vi "HRV_EEG_version2.vi"() -> ()   [LabVIEW 2014]
uses:
  <vilib>/Utility/file.llb/Read From Spreadsheet File (I64).vi
panel:
  out "PPI+ERP":dbl[][](graph)
  out "HF+ERP":dbl[][](graph)
  out "LF+ERP":dbl[][](graph)
  out "VLF+ERP":dbl[][](graph)
  out "PPI":dbl[][](graph)
  in  "PPI":path=path "C:/Users/Jaehong/Desktop/Classifiers/HRV_EEG/LF Maker/김다영_PPI.txt"
  in  "HF":path=path "C:/Users/Jaehong/Desktop/Classifiers/HRV_EEG/LF Maker/김다영_HF.txt"
  in  "LF":path=path "C:/Users/Jaehong/Desktop/Classifiers/HRV_EEG/LF Maker/김다영_LF.txt"
  in  "VLF":path=path "C:/Users/Jaehong/Desktop/Classifiers/HRV_EEG/LF Maker/김다영_VLF.txt"
  in  "강제 Execution":bool
  out "HF":dbl[][](graph)
  out "LF":dbl[][](graph)
  out "VLF":dbl[][](graph)
  out "Executing":bool
  out "Target_icon":i64
  in  "Target_Total":path=path "C:/Users/Jaehong/Desktop/Classifiers/data/통합LDAs/김다영/target_order.txt"
  in  "Icon_number":i32=1
  out "ERP_Graph":dbl[][](graph)
  in  "Trial_Number":i32=1
  in  "ERP_Total":path=path "C:/Users/Jaehong/Desktop/Classifiers/HRV_EEG/ERP_total/김다영/ERP_total.txt"
  in  "stop":bool
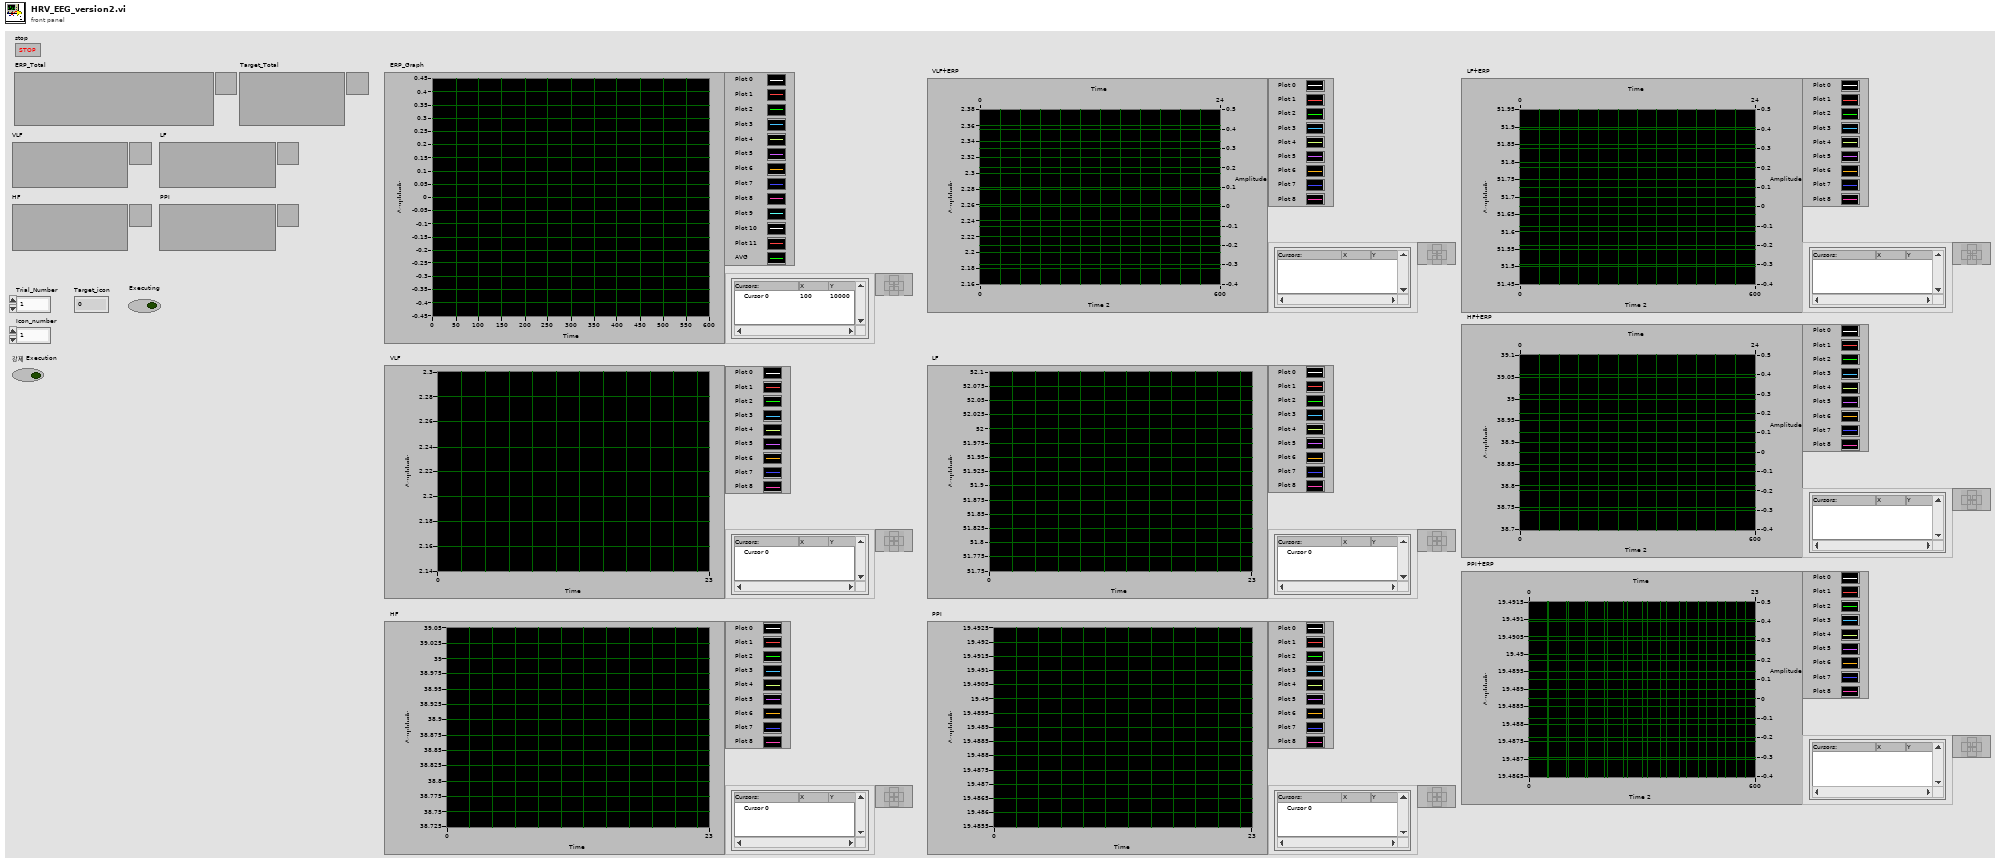
[diagram p1: front panel]
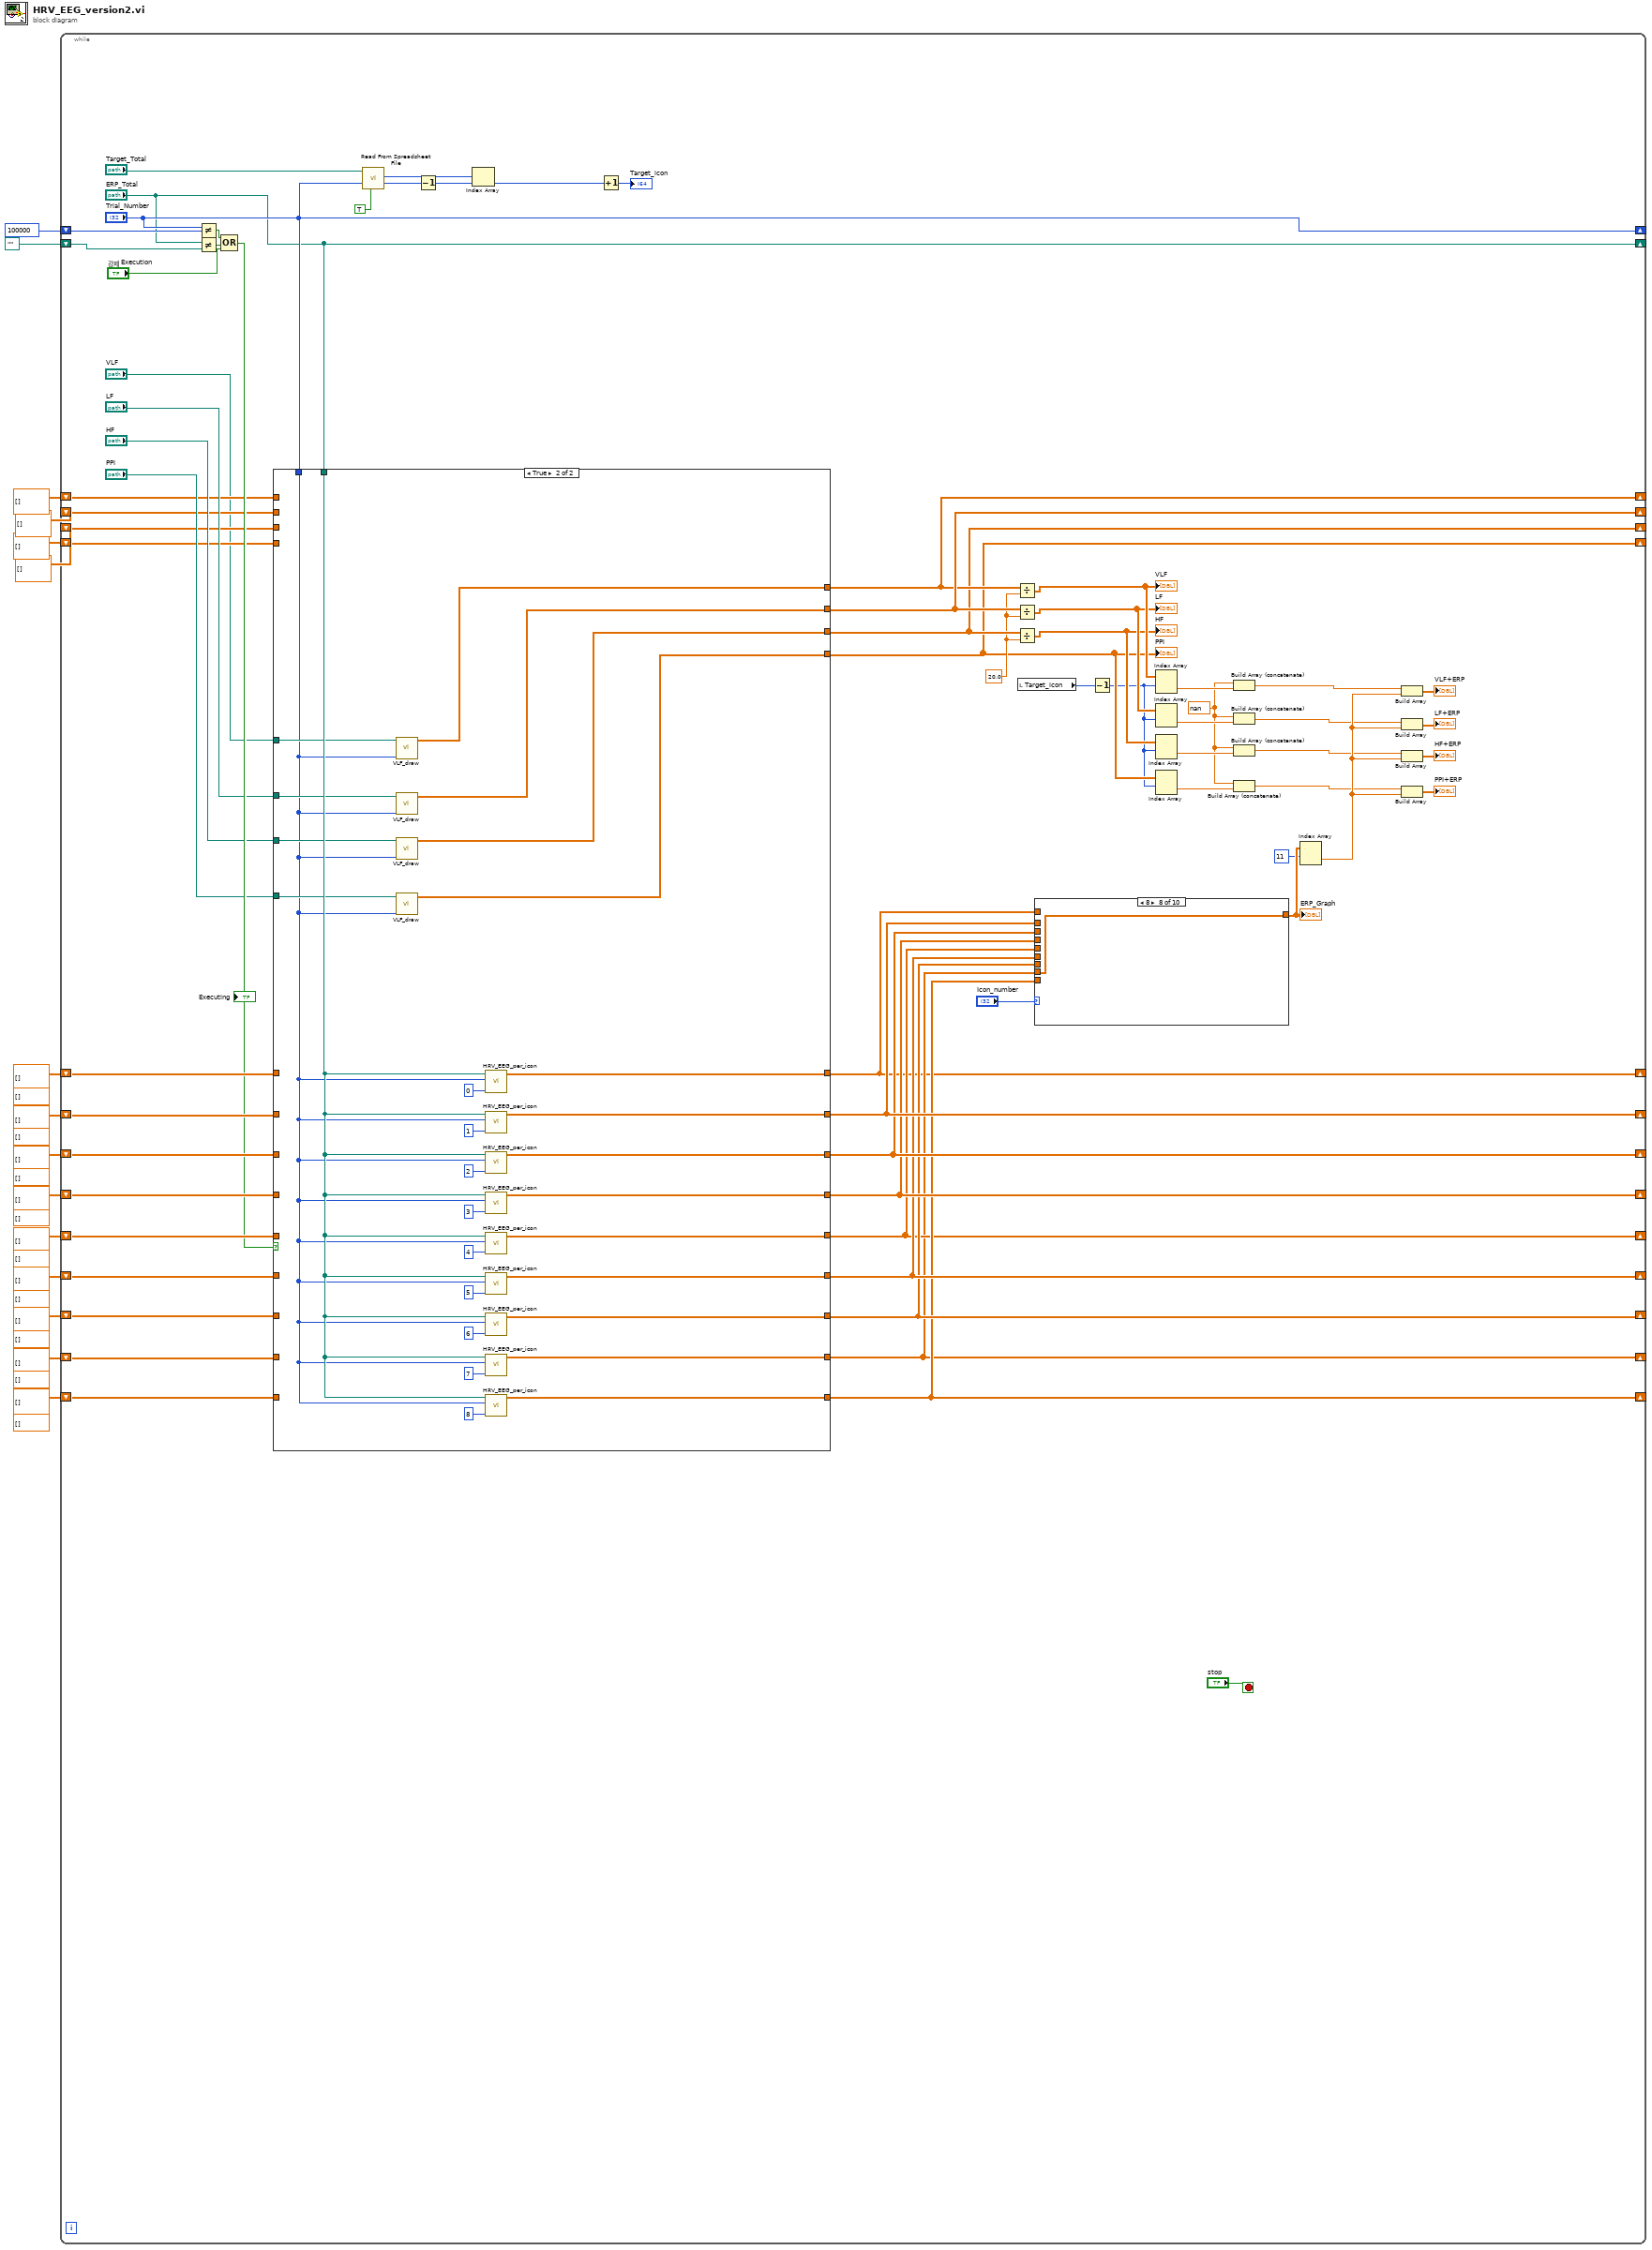
[diagram p0: block diagram]
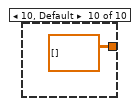
[diagram p11: hidden frame]
diagram:
  (unwired) dbl[] [] ("PRV% (VLF, LF, HF)")
  (unwired) dbl[] [] ("PRV% (VLF, LF, HF)")
  (unwired) dbl[] [] ("PRV% (VLF, LF, HF)")
  (unwired) dbl[] [] ("PRV% (VLF, LF, HF)")
  (unwired) dbl[] [] ("PRV% (VLF, LF, HF)")
  (unwired) dbl[] [] ("PRV% (VLF, LF, HF)")
  (unwired) dbl[] [] ("PRV% (VLF, LF, HF)")
  (unwired) dbl[] [] ("PRV% (VLF, LF, HF)")
  (unwired) dbl[] [] ("PRV% (VLF, LF, HF)")
  n1 = while {
    shift-right: [w39] -> _
    shift-left: dbl[][] [] ("Icon1") -> [w72]
    shift-right: [w78] -> _
    shift-left: dbl[][] [] ("Icon1") -> [w71]
    shift-right: [w77] -> _
    shift-left: dbl[][] [] ("Icon1") -> [w70]
    shift-right: [w76] -> _
    shift-left: dbl[][] [] ("Icon1") -> [w69]
    shift-right: [w57] -> _
    shift-left: dbl[][] [] ("Icon1") -> [w68]
    shift-right: [w75] -> _
    shift-left: dbl[][] [] ("Icon1") -> [w67]
    shift-right: [w74] -> _
    shift-left: dbl[][] [] ("Icon1") -> [w66]
    shift-right: [w56] -> _
    shift-left: dbl[][] [] ("Icon1") -> [w65]
    shift-right: [w73] -> _
    shift-left: dbl[][] [] ("Icon1") -> [w64]
    shift-right: ["Trial_Number"] -> _
    shift-left: 100000 -> [w63]
    shift-right: ["ERP_Total"] -> _
    shift-left: path "" ("ERP_Total") -> [w60]
    shift-right: [w43] -> _
    shift-left: dbl[][] [] ("Icon1") -> [w48]
    shift-right: [w49] -> _
    shift-left: dbl[][] [] ("Icon1") -> [w47]
    shift-right: [w42] -> _
    shift-left: dbl[][] [] ("Icon1") -> [w46]
    shift-right: [w33] -> _
    shift-left: dbl[][] [] ("Icon1") -> [w45]
    stop <- "stop" stop-if-true
    w17 = nan
    w41 = 20.0
    n2 = Not Equal?(x="Trial_Number", y=w63) -> (x != y?=w59:bool)
    n3 = Not Equal?(x="ERP_Total", y=w60) -> (x != y?=w55:bool)
    n4 = Compound Arithmetic op=OR(w59, w55, "강제 Execution") -> (w58:bool)
    "Executing" <- w58
    n5 = case shown="True" w58 {
      tunnel: "ERP_Total" -> [_ w106]
      tunnel: "Trial_Number" -> [_ w101]
      tunnel: [w96 w115] -> w39
      tunnel: [w95 w114] -> w78
      tunnel: [w94 w113] -> w77
      tunnel: [w93 w112] -> w76
      tunnel: [w92 w111] -> w57
      tunnel: [w91 w110] -> w75
      tunnel: [w90 w109] -> w74
      tunnel: [w89 w108] -> w56
      tunnel: [w88 w107] -> w73
      tunnel: w72 -> [w96 _]
      tunnel: w71 -> [w95 _]
      tunnel: w70 -> [w94 _]
      tunnel: w69 -> [w93 _]
      tunnel: w68 -> [w92 _]
      tunnel: w67 -> [w91 _]
      tunnel: w66 -> [w90 _]
      tunnel: w65 -> [w89 _]
      tunnel: w64 -> [w88 _]
      tunnel: "VLF" -> [_ w105]
      tunnel: "LF" -> [_ w104]
      tunnel: "HF" -> [_ w103]
      tunnel: "PPI" -> [_ w102]
      tunnel: [w87 w100] -> w43
      tunnel: [w86 w99] -> w49
      tunnel: [w85 w98] -> w42
      tunnel: [w84 w97] -> w33
      tunnel: w48 -> [w87 _]
      tunnel: w47 -> [w86 _]
      tunnel: w46 -> [w85 _]
      tunnel: w45 -> [w84 _]
      frame False {
      }
      frame True {
        n6 = call "VLF_draw.vi"("Trial_Number"=w101, "HRV(VLF, LF, HF, PPI)"=w105) -> ("Icon1"=w100:dbl[][])  [unwired: 9 in]
        n7 = call "VLF_draw.vi"("Trial_Number"=w101, "HRV(VLF, LF, HF, PPI)"=w104) -> ("Icon1"=w99:dbl[][])  [unwired: 9 in]
        n8 = call "VLF_draw.vi"("Trial_Number"=w101, "HRV(VLF, LF, HF, PPI)"=w103) -> ("Icon1"=w98:dbl[][])  [unwired: 9 in]
        n9 = call "VLF_draw.vi"("Trial_Number"=w101, "HRV(VLF, LF, HF, PPI)"=w102) -> ("Icon1"=w97:dbl[][])  [unwired: 9 in]
        n10 = call "HRV_EEG_per_icon.vi"("Icon Number"=0, "Trial_Number"=w101, "ERP_Total"=w106) -> ("Icon1"=w115:dbl[][])  [unwired: 8 in]
        n11 = call "HRV_EEG_per_icon.vi"("Icon Number"=1, "Trial_Number"=w101, "ERP_Total"=w106) -> ("Icon1"=w114:dbl[][])  [unwired: 8 in]
        n12 = call "HRV_EEG_per_icon.vi"("Icon Number"=2, "Trial_Number"=w101, "ERP_Total"=w106) -> ("Icon1"=w113:dbl[][])  [unwired: 8 in]
        n13 = call "HRV_EEG_per_icon.vi"("Icon Number"=3, "Trial_Number"=w101, "ERP_Total"=w106) -> ("Icon1"=w112:dbl[][])  [unwired: 8 in]
        n14 = call "HRV_EEG_per_icon.vi"("Icon Number"=4, "Trial_Number"=w101, "ERP_Total"=w106) -> ("Icon1"=w111:dbl[][])  [unwired: 8 in]
        n15 = call "HRV_EEG_per_icon.vi"("Icon Number"=5, "Trial_Number"=w101, "ERP_Total"=w106) -> ("Icon1"=w110:dbl[][])  [unwired: 8 in]
        n16 = call "HRV_EEG_per_icon.vi"("Icon Number"=6, "Trial_Number"=w101, "ERP_Total"=w106) -> ("Icon1"=w109:dbl[][])  [unwired: 8 in]
        n17 = call "HRV_EEG_per_icon.vi"("Icon Number"=7, "Trial_Number"=w101, "ERP_Total"=w106) -> ("Icon1"=w108:dbl[][])  [unwired: 8 in]
        n18 = call "HRV_EEG_per_icon.vi"("Icon Number"=8, "Trial_Number"=w101, "ERP_Total"=w106) -> ("Icon1"=w107:dbl[][])  [unwired: 8 in]
      }
    }
    "PPI" <- w33
    n19 = call-poly <vilib>:"Read From Spreadsheet File.vi"("transpose (no:F)"=TRUE, "file path (dialog if empty)"="Target_Total") -> ("first row"=w80:i64[])  [unwired: 5 in, 4 out]
    n20 = Decrement(x="Trial_Number") -> (x-1=w40:i32)
    n21 = Index Array(array=w80, index=w40) -> (element=w79:i64)
    n22 = Increment(x=w79) -> (x+1=→"Target_icon":i64)
    n23 = Divide(x=w43, y=w41) -> (x/y=w36:dbl[][])
    "VLF" <- w36
    n24 = Divide(x=w49, y=w41) -> (x/y=w35:dbl[][])
    "LF" <- w35
    n25 = Divide(x=w42, y=w41) -> (x/y=w34:dbl[][])
    "HF" <- w34
    n26 = local read "Target_icon"() -> (w32:i64)
    n27 = case shown="8" "Icon_number" {
      tunnel: w39 -> [w125 _ _ _ _ _ _ _ _ _]
      tunnel: w78 -> [_ w126 _ _ _ _ _ _ _ _]
      tunnel: w77 -> [_ _ w127 _ _ _ _ _ _ _]
      tunnel: w76 -> [_ _ _ w128 _ _ _ _ _ _]
      tunnel: w57 -> [_ _ _ _ w129 _ _ _ _ _]
      tunnel: w75 -> [_ _ _ _ _ w130 _ _ _ _]
      tunnel: w74 -> [_ _ _ _ _ _ w131 _ _ _]
      tunnel: w56 -> [_ _ _ _ _ _ _ w132 _ _]
      tunnel: w73 -> [_ _ _ _ _ _ _ _ w133 _]
      tunnel: [w125 w126 w127 w128 w129 w130 w131 w132 w133 dbl[][] [] ("Icon1")] -> w38
      frame 1 {
      }
      frame 2 {
      }
      frame 3 {
      }
      frame 4 {
      }
      frame 5 {
      }
      frame 6 {
      }
      frame 7 {
      }
      frame 8 {
      }
      frame 9 {
      }
      frame 10, Default {
      }
    }
    "ERP_Graph" <- w38
    n28 = Decrement(x=w32) -> (x-1=w31:i64)
    n29 = Index Array(array=w36, index (row)=w31) -> (element=w29:dbl[])  [unwired: 1 in]
    n30 = Index Array(array=w35, index (row)=w31) -> (element=w28:dbl[])  [unwired: 1 in]
    n31 = Index Array(array=w34, index (row)=w31) -> (element=w27:dbl[])  [unwired: 1 in]
    n32 = Index Array(array=w33, index (row)=w31) -> (element=w26:dbl[])  [unwired: 1 in]
    n33 = Build Array (concatenate)(w17, w29) -> (w21:dbl[])
    n34 = Build Array (concatenate)(w17, w28) -> (w20:dbl[])
    n35 = Build Array (concatenate)(w17, w27) -> (w19:dbl[])
    n36 = Build Array (concatenate)(w17, w26) -> (w18:dbl[])
    n37 = Index Array(array=w38, index (row)=11) -> (element=w25:dbl[])  [unwired: 1 in]
    n38 = Build Array(w21, w25) -> (→"VLF+ERP":dbl[][])
    n39 = Build Array(w20, w25) -> (→"LF+ERP":dbl[][])
    n40 = Build Array(w19, w25) -> (→"HF+ERP":dbl[][])
    n41 = Build Array(w18, w25) -> (→"PPI+ERP":dbl[][])
  }
